vi "Timed Write to Hardware.vi"(7 "Valid":bool, 8 "error in (no error)":errorcluster, 9 "Trigger Values":dbl[](array[numeric]), 10 "Values":dbl[](array[numeric]), 11 "Execution Unit in":refnum<class "Execution Unit.lvclass">) -> (0 "error out":errorcluster, 1 "Trigger Values out":dbl[](array[numeric]), 2 "Values out":dbl[](array[numeric]), 3 "Execution Unit out":refnum<class "Execution Unit.lvclass">)   [LabVIEW 2020, in "AIM ARINC 429 Engine.lvlib" / "Custom Device.lvlib"]
uses:
  Custom Device.lvlib
  Interfaces/Execution Unit/Execution Unit.lvclass
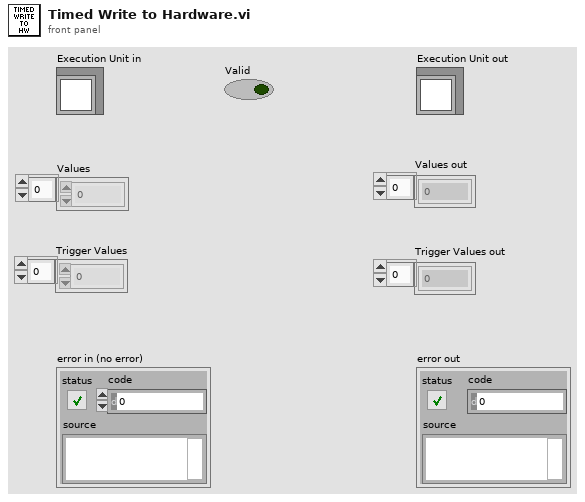
[diagram p1: front panel]
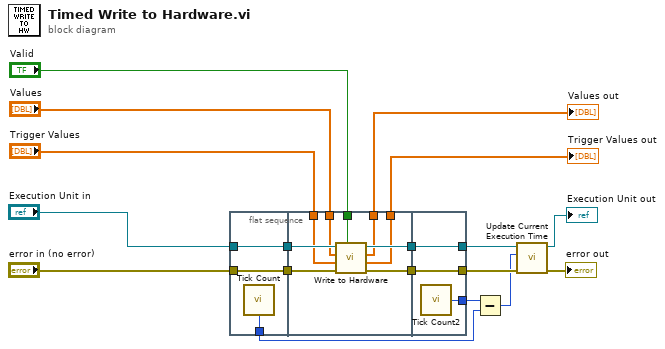
[diagram p0: block diagram]
diagram:
  n1 = flat-sequence {
    tunnel: "error in (no error)" -> [w20]
    tunnel: "Execution Unit in" -> [w21]
    tunnel: [w21] -> w18
    tunnel: [w20] -> w17
    tunnel: [w19] -> w14
    tunnel: "Valid" -> [w28]
    tunnel: w18 -> [w30]
    tunnel: w17 -> [w29]
    tunnel: [w27] -> w16
    tunnel: [w26] -> w15
    tunnel: [w25] -> w9
    tunnel: [w24] -> w8
    tunnel: "Values" -> [w23]
    tunnel: "Trigger Values" -> [w22]
    tunnel: [w32] -> w5
    tunnel: [w33] -> w4
    tunnel: w16 -> [w33]
    tunnel: w15 -> [w32]
    tunnel: [w31] -> w13
    frame #0 {
      n2 = call "Tick Count"() -> ("Tick Count(uSec)"=w19:u32)
    }
    frame #1 {
      n3 = call-dynamic "Write to Hardware.vi"("Valid Triggers"=w28, "error in (no error)"=w29, "Trigger Values"=w22, "Values in"=w23, "Execution Unit in"=w30) -> ("error out"=w26:errorcluster, "Trigger Values out"=w24:dbl[], "Values out"=w25:dbl[], "Execution Unit out"=w27:refnum<class "Execution Unit.lvclass">)  [unwired: 3 in]
    }
    frame #2 {
      n4 = call "Tick Count2"() -> ("Tick Count(uSec)"=w31:u32)
    }
  }
  n5 = Subtract(x=w13, y=w14) -> (x-y=w1:u32)
  n6 = call-dynamic "Update Current Execution Time.vi"("error in (no error)"=w5, "Current Execution Time (us)"=w1, "Execution Unit in"=w4) -> ("error out"=→"error out":errorcluster, "Execution Unit out"=→"Execution Unit out":refnum<class "Execution Unit.lvclass">)  [unwired: 7 in]
  "Values out" <- w9
  "Trigger Values out" <- w8
